vi "Start Connection Listener.vi"(8 "error in (no error)":errorcluster, 10 "Timeout (-1)":i32=-1, 11 "Websocket In":refnum<class "Websocket.lvclass">) -> (0 "error out":errorcluster, 2 "Timed Out":bool, 3 "Websocket Out":refnum<class "Websocket.lvclass">)   [LabVIEW 2017, in "Front Panel Publisher.lvlib" / "Websocket.lvclass"]
doc: "Looks up an existing object matching object name or creates a new object and returns a refnum you can use when calling other class methods.\n\nObjects created with this VI should be destroyed using this class Delete VI."
uses:
  Websocket.lvclass
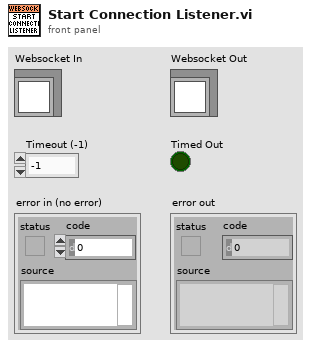
[diagram p1: front panel]
types:
  T1 = enum16{"ReadRepository", "CreateNew", "CreateOrLookUpExisting", "ReadRepositoryAndDestroy"}
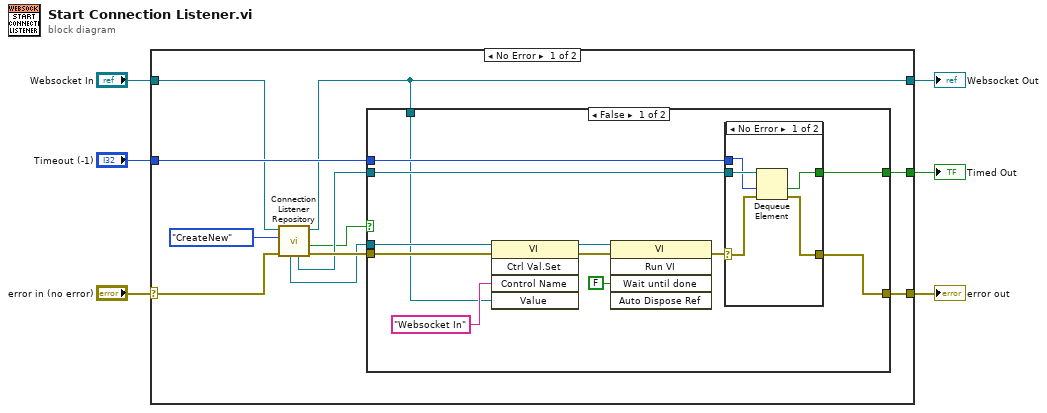
[diagram p0: block diagram]
diagram:
  n1 = case shown="No Error" "error in (no error)" {
    selector: "error in (no error)" -> [w14 w37]
    tunnel: [w15 w37] -> w5
    tunnel: [w10 w38] -> w3
    tunnel: "Websocket In" -> [w8 w38]
    tunnel: "Timeout (-1)" -> [w17 _]
    tunnel: [w16 _] -> w1
    frame No Error {
      n2 = call "Connection Listener Repository.vi"("error in (no error)"=w14, "Action(ReadRepository)"=T1."CreateNew", "Websocket In"=w8) -> ("error out"=w13:errorcluster, "ProcessAlreadyStarted"=w9:bool, "Websocket Out"=w10:refnum<class "Websocket.lvclass">, "ProcessSyncQueue"=w11:refnum<queue>, "ProcessViRef"=w12:refnum<vi>)  [unwired: 2 in, 2 out]
      n3 = case shown="False" w9 {
        tunnel: w17 -> [w25 _]
        tunnel: [w24 _] -> w16
        tunnel: [w22 w36] -> w15
        tunnel: w13 -> [w21 w36]
        tunnel: w12 -> [w20 _]
        tunnel: w11 -> [w19 _]
        tunnel: w10 -> [w18 _]
        frame False {
          n4 = invoke class="VI" method="Ctrl Val.Set"(reference=w20, error in=w21, "Control Name"="Websocket In", "Value"=w18) -> (reference out=w28:refnum<vi>, error out=w27:errorcluster)  [unwired: 1 in, 3 out]
          n5 = invoke class="VI" method="Run VI"(reference=w28, error in=w27, "Wait until done"=FALSE ("Wait Until Done")) -> (error out=w23:errorcluster)  [unwired: 2 in, 4 out]
          n6 = case shown="No Error" w23 {
            tunnel: w19 -> [w34 _]
            tunnel: w25 -> [w32 _]
            tunnel: [w33 _] -> w24
            selector: w23 -> [w31 w35]
            tunnel: [w30 w35] -> w22
            frame No Error {
              n7 = Dequeue Element(queue=w34, timeout in ms (-1)=w32, error in (no error)=w31) -> (timed out?=w33:bool, error out=w30:errorcluster)  [unwired: 2 out]
            }
            frame Error {
            }
          }
        }
        frame True {
          # "Process Already started.\nThis option will only be used togeather with the\naction: \"CreateOrLookUpExisting\""
        }
      }
    }
    frame Error {
    }
  }
  "error out" <- w5
  "Websocket Out" <- w3
  "Timed Out" <- w1
